vi "Lorentzian-Fitter v1.vi"() -> ()   [LabVIEW 2014]
uses:
  <vilib>/Utility/file.llb/Read From Spreadsheet File (DBL).vi
  <vilib>/gmath/NumericalOptimization/Nonlinear Curve Fit LM bound.vi
  <vilib>/gmath/NI_Gmath.lvlib
panel:
  out "best fit params":dbl[](array[numeric])
  out "initial params":dbl[](array[numeric])
  out "Subset and Fit":cluster{dbl[], "best nonlinear fit":dbl[]}[](graph)
  out "Data and bg":cluster{"all rows":dbl[], "all rows":dbl[]}[](graph)
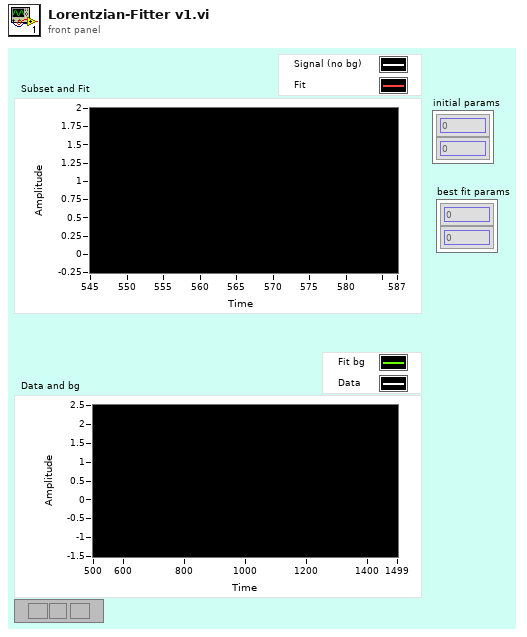
[diagram p1: front panel]
types:
  T1 = cluster{"parameter minimum":dbl[], "parameter maximum":dbl[]}
  T2 = typedef "eventvkey.ctl" = enum16{"ASCII", "Enter", "Return", "Shift", "Ctrl", "Alt", "Cmd", "Opt", "Caps", "NumLock", "Clear", "Break", "Up", "Down", "Left", "Right", "Insert", "Delete", "Home", "End", "PageUp", "PageDown", "Escape", "Help", "Pause", "ScrollLock", "F1", "F2", "F3", "F4", "F5", "F6", "F7", "F8", "F9", "F10", "F11", "F12", "F13", "F14", "F15", "F16", "F17", "F18", "F19", "F20", "F21", "F22", "F23", "F24", "Play", "VolumeUp", "VolumeDown", "Mute", "Two Byte Char"}
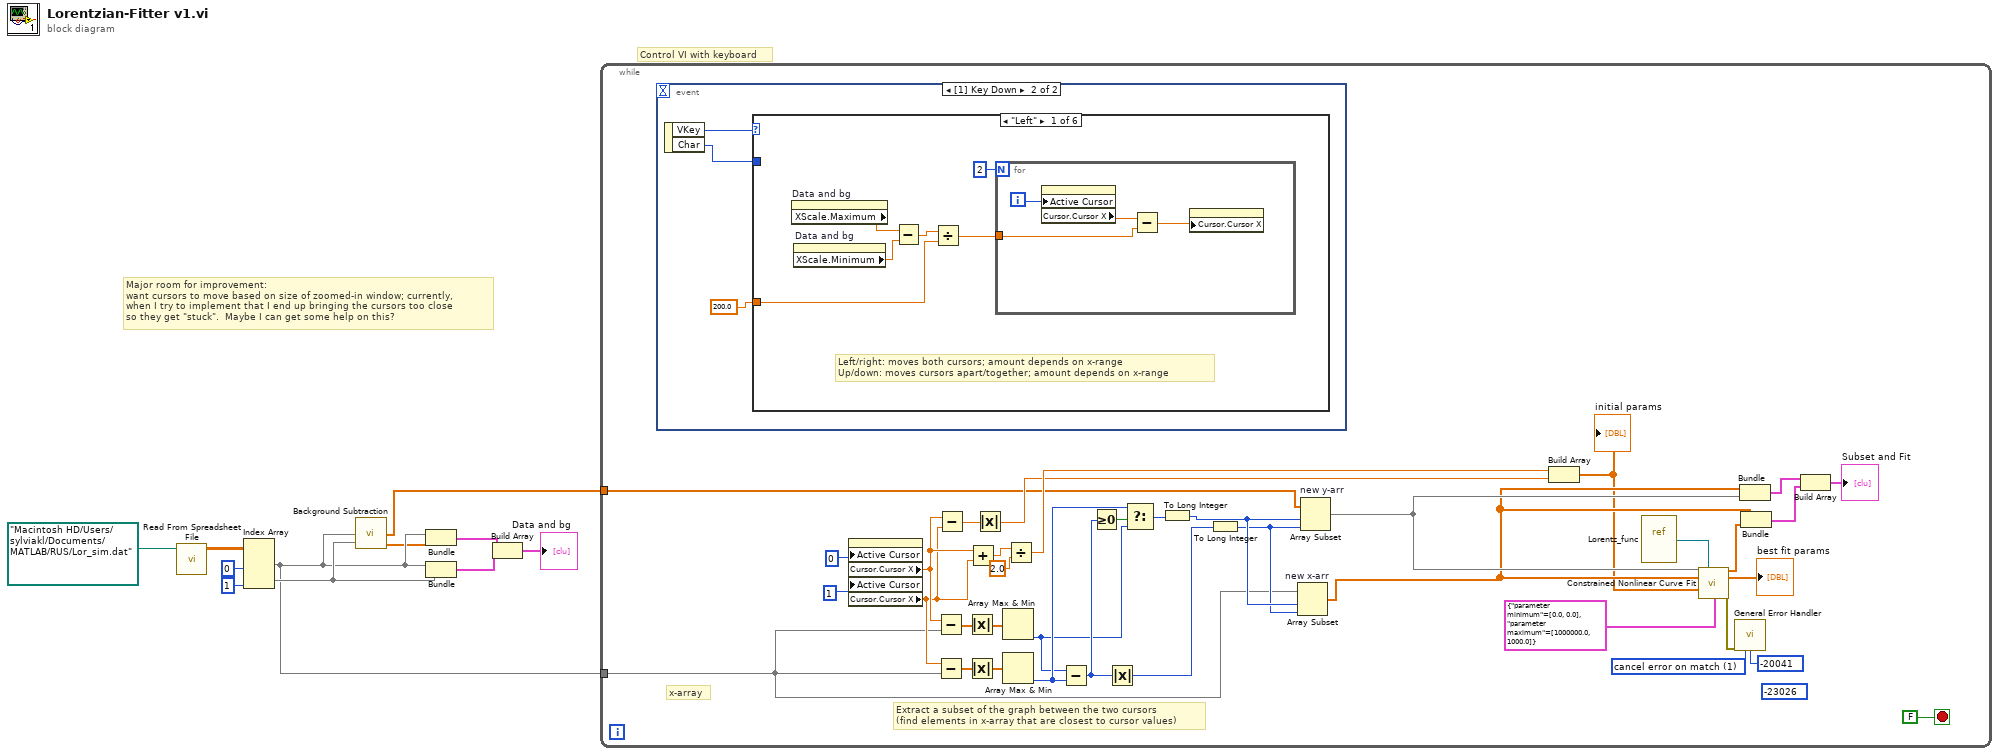
[diagram p0: block diagram]
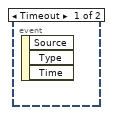
[diagram p2: hidden frame]
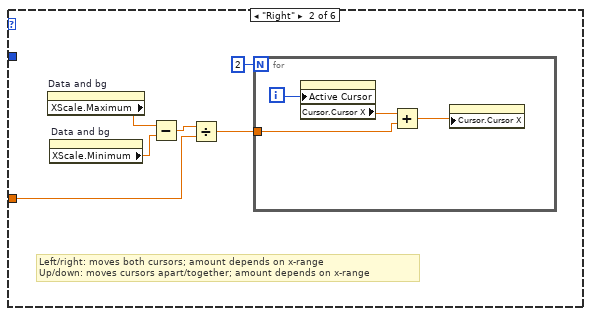
[diagram p3: hidden frame]
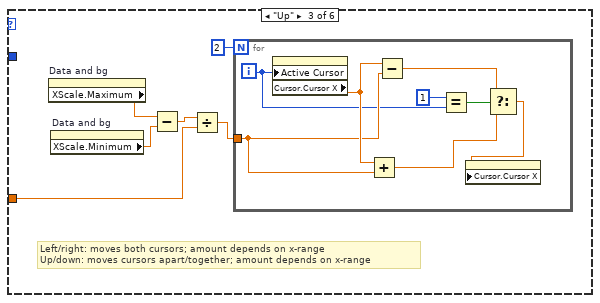
[diagram p4: hidden frame]
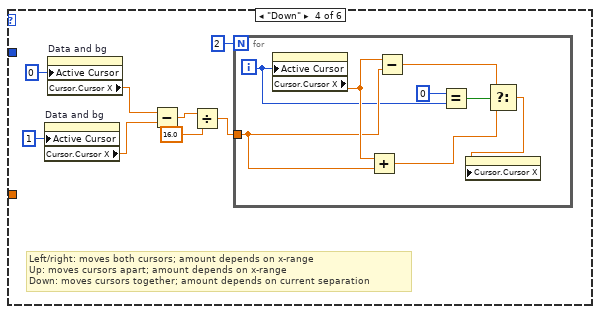
[diagram p5: hidden frame]
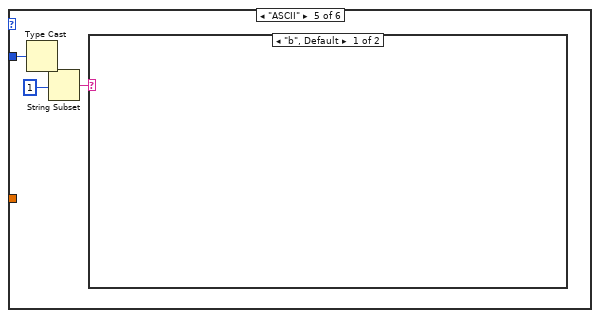
[diagram p6: hidden frame]
diagram:
  # "Major room for improvement:\nwant cursors to move based on size of zoomed-in window; currently,\nwhen I try to implement that I end up bringing the cursors too close\nso they get \"stuck\".  Maybe I can get some help on this?"
  # "Control VI with keyboard"
  n1 = call-poly <vilib>:"Read From Spreadsheet File.vi"("file path (dialog if empty)"=path "/Macintosh HD/Users/sylviakl/Documents/MATLAB/RUS/Lor_sim.dat") -> ("all rows"=w8:dbl[][])  [unwired: 6 in, 4 out]
  n2 = Index Array(array=w8, index (col) #1=0 ("disabled index (col)"), index (col) #2=1 ("index (col)")) -> (element #1=w6:dbl[], element #2=w7:dbl[])  [unwired: 2 in]
  n3 = call "Background Subtraction.vi"("X"=w6, "Y"=w7) -> ("signal"=w2:dbl[], "background"=w1:dbl[])  [unwired: 1 out]
  n4 = Bundle("all rows"=w6, "background"=w1) -> (w5:cluster{"all rows":dbl[], "background":dbl[]})  [unwired: 1 in]
  n5 = Bundle("all rows"=w6, "all rows"=w7) -> (w4:cluster{"all rows":dbl[], "all rows":dbl[]})  [unwired: 1 in]
  n6 = Build Array(w5, w4) -> (→"Data and bg":cluster{"all rows":dbl[], "all rows":dbl[]}[])
  n7 = while {
    tunnel: w6 -> [w14]
    tunnel: w2 -> [w13]
    stop <- FALSE stop-if-true
    (unwired) -23026 ("[exception code]")
    w18 = 1 items=["no exception", "cancel error on match", "set error on match"] ("[exception action] (none:0)")
    # "x-array"
    # "Extract a subset of the graph between the two cursors\n(find elements in x-array that are closest to cursor values)"
    n8 = event shown="[1] Key Down" {
      selector: _ -> [_ _]
      dyn-events: _ -> [_ _]
      timeout: _ -> [_ _]
      event Timeout {
        n9 = event-data() -> ()  [unwired: 1 in, 3 out]
      }
      event Key Down {
        n10 = event-data() -> ("VKey"=w51:T2, "Char"=w50:i16)  [unwired: 1 in]
        n11 = case shown="\"Left\"" w51 {
          tunnel: w50 -> [_ _ _ _ w105 _]
          tunnel: 200.0 ("y") -> [w52 w62 w72 _ _ _]
          frame "Left" {
            # "Left/right: moves both cursors; amount depends on x-range\nUp/down: moves cursors apart/together; amount depends on x-range"
            n12 = property on="Data and bg" class="XYGraph (strict)"() -> ("XScale.Maximum"=w55:dbl)  [unwired: 2 in, 2 out]
            n13 = property on="Data and bg" class="XYGraph (strict)"() -> ("XScale.Minimum"=w54:dbl)  [unwired: 2 in, 2 out]
            n14 = Subtract(x=w55, y=w54) -> (x-y=w56:dbl)
            n15 = Divide(x=w56, y=w52) -> (x/y=w53:dbl)
            n16 = for {
              N: 2 -> [_]
              tunnel: w53 -> [w58]
              i -> [w59]
              n17 = property on="Data and bg" class="XYGraph (strict)"("Active Cursor"=w59) -> ("Cursor.Cursor X"=w60:dbl)  [unwired: 2 in, 2 out]
              n18 = Subtract(x=w60, y=w58) -> (x-y=w61:dbl)
              n19 = property on="Data and bg" class="XYGraph (strict)"("Cursor.Cursor X"=w61) -> ()  [unwired: 2 in, 2 out]
            }
          }
          frame "Right" {
            # "Left/right: moves both cursors; amount depends on x-range\nUp/down: moves cursors apart/together; amount depends on x-range"
            n20 = property on="Data and bg" class="XYGraph (strict)"() -> ("XScale.Maximum"=w65:dbl)  [unwired: 2 in, 2 out]
            n21 = property on="Data and bg" class="XYGraph (strict)"() -> ("XScale.Minimum"=w64:dbl)  [unwired: 2 in, 2 out]
            n22 = Subtract(x=w65, y=w64) -> (x-y=w66:dbl)
            n23 = Divide(x=w66, y=w62) -> (x/y=w63:dbl)
            n24 = for {
              N: 2 -> [_]
              tunnel: w63 -> [w68]
              i -> [w69]
              n25 = property on="Data and bg" class="XYGraph (strict)"("Active Cursor"=w69) -> ("Cursor.Cursor X"=w70:dbl)  [unwired: 2 in, 2 out]
              n26 = Add(x=w70, y=w68) -> (x+y=w71:dbl)
              n27 = property on="Data and bg" class="XYGraph (strict)"("Cursor.Cursor X"=w71) -> ()  [unwired: 2 in, 2 out]
            }
          }
          frame "Up" {
            # "Left/right: moves both cursors; amount depends on x-range\nUp/down: moves cursors apart/together; amount depends on x-range"
            n28 = property on="Data and bg" class="XYGraph (strict)"() -> ("XScale.Maximum"=w75:dbl)  [unwired: 2 in, 2 out]
            n29 = property on="Data and bg" class="XYGraph (strict)"() -> ("XScale.Minimum"=w74:dbl)  [unwired: 2 in, 2 out]
            n30 = Subtract(x=w75, y=w74) -> (x-y=w76:dbl)
            n31 = Divide(x=w76, y=w72) -> (x/y=w73:dbl)
            n32 = for {
              N: 2 -> [_]
              tunnel: w73 -> [w84]
              i -> [w79]
              n33 = property on="Data and bg" class="XYGraph (strict)"("Active Cursor"=w79) -> ("Cursor.Cursor X"=w85:dbl)  [unwired: 2 in, 2 out]
              n34 = Add(x=w85, y=w84) -> (x+y=w82:dbl)
              n35 = Subtract(x=w85, y=w84) -> (x-y=w83:dbl)
              n36 = Equal?(x=1, y=w79) -> (x = y?=w80:bool)
              n37 = Select(t=w83, s=w80, f=w82) -> (s? t:f=w81:dbl)
              n38 = property on="Data and bg" class="XYGraph (strict)"("Cursor.Cursor X"=w81) -> ()  [unwired: 2 in, 2 out]
            }
          }
          frame "Down" {
            # "Left/right: moves both cursors; amount depends on x-range\nUp: moves cursors apart; amount depends on x-range\nDown: moves cursors together; amount depends on current separation"
            n39 = property on="Data and bg" class="XYGraph (strict)"("Active Cursor"=u32 1) -> ("Cursor.Cursor X"=w89:dbl)  [unwired: 2 in, 2 out]
            n40 = property on="Data and bg" class="XYGraph (strict)"("Active Cursor"=u32 0) -> ("Cursor.Cursor X"=w88:dbl)  [unwired: 2 in, 2 out]
            n41 = Subtract(x=w88, y=w89) -> (x-y=w92:dbl)
            n42 = Divide(x=w92, y=16.0) -> (x/y=w91:dbl)
            n43 = for {
              N: 2 -> [_]
              tunnel: w91 -> [w100]
              i -> [w95]
              n44 = property on="Data and bg" class="XYGraph (strict)"("Active Cursor"=w95) -> ("Cursor.Cursor X"=w101:dbl)  [unwired: 2 in, 2 out]
              n45 = Add(x=w101, y=w100) -> (x+y=w98:dbl)
              n46 = Subtract(x=w101, y=w100) -> (x-y=w99:dbl)
              n47 = Equal?(x=0, y=w95) -> (x = y?=w96:bool)
              n48 = Select(t=w99, s=w96, f=w98) -> (s? t:f=w97:dbl)
              n49 = property on="Data and bg" class="XYGraph (strict)"("Cursor.Cursor X"=w97) -> ()  [unwired: 2 in, 2 out]
            }
          }
          frame "ASCII" {
            n50 = Type Cast(x=w105) -> (*(type *) &x=w104:string)  [unwired: 1 in]
            n51 = String Subset(string=w104, offset (0)=1) -> (substring=w102:string)  [unwired: 1 in]
            n52 = case shown="\"b\", Default" w102 {
              frame "b", Default {
              }
              frame "a" {
              }
            }
          }
          frame Default {
          }
        }
      }
    }
    n53 = property on="Data and bg" class="XYGraph (strict)"("Active Cursor"=u32 0, "Active Cursor"=u32 1) -> ("Cursor.Cursor X"=w30:dbl, "Cursor.Cursor X"=w29:dbl)  [unwired: 2 in, 2 out]
    n54 = Subtract(x=w30, y=w14) -> (x-y=w43:dbl[])
    n55 = Subtract(x=w29, y=w14) -> (x-y=w45:dbl[])
    n56 = Subtract(x=w30, y=w29) -> (x-y=w28:dbl)
    n57 = Absolute Value(x=w43) -> (abs(x)=w42:dbl[])
    n58 = Absolute Value(x=w45) -> (abs(x)=w44:dbl[])
    n59 = Add(x=w30, y=w29) -> (x+y=w33:dbl)
    n60 = Absolute Value(x=w28) -> (abs(x)=w27:dbl)
    n61 = Array Max & Min(array=w42) -> (min index (indices)=w34:i32)  [unwired: 3 out]
    n62 = Array Max & Min(array=w44) -> (min index (indices)=w35:i32)  [unwired: 3 out]
    n63 = Divide(x=w33, y=2.0) -> (x/y=w31:dbl)
    n64 = Subtract(x=w34, y=w35) -> (x-y=w39:i32)
    n65 = Greater Or Equal To 0?(x=w39) -> (x >= 0?=w38:bool)
    n66 = Absolute Value(x=w39) -> (abs(x)=w41:i32)
    n67 = Select(t=w35, s=w38, f=w34) -> (s? t:f=w40:i32)
    n68 = To Long Integer(number=w40) -> (32bit integer=w37:i32)
    n69 = To Long Integer(number=w41) -> (32bit integer=w36:i32)
    n70 = Array Subset "new x-arr"(array=w14, index=w37, length=w36) -> (w21:dbl[])
    n71 = Array Subset "new y-arr"(array=w13, index=w37, length=w36) -> (w22:dbl[])
    n72 = Build Array(w31, w27) -> (w20:dbl[])
    "initial params" <- w20
    n73 = vi-ref "Lorentz_func.vi"() -> (w23:refnum<vi>)
    n74 = call-poly <vilib>:"Constrained Nonlinear Curve Fit.vi"("Y"=w22, "f(x,a)"=w23, "X"=w21, "initial parameters"=w20, "parameter bounds"=T1 {"parameter minimum"=[0.0, 0.0], "parameter maximum"=[1000000.0, 1000.0]}) -> ("best nonlinear fit"=w17:dbl[], "best fit parameters"=→"best fit params":dbl[], "error out"=w15:errorcluster)  [unwired: 5 in, 3 out]
    n75 = call <vilib>:"General Error Handler.vi"("error in (no error)"=w15, "[exception action] (none:0)"=w18, "[exception code]"=-20041) -> ()  [unwired: 8 in, 5 out]
    n76 = Bundle(w21, w22) -> (w25:cluster{dbl[], dbl[]})  [unwired: 1 in]
    n77 = Bundle(w21, "best nonlinear fit"=w17) -> (w24:cluster{dbl[], "best nonlinear fit":dbl[]})  [unwired: 1 in]
    n78 = Build Array(w25, w24) -> (→"Subset and Fit":cluster{dbl[], "best nonlinear fit":dbl[]}[])
  }
